vi "GetRectangles.vi"(0 "reference in":refnum<class "Pgui_Obj.lvclass">, 5 "error in (no error)":errorcluster) -> (14 "reference out":refnum<class "Pgui_Obj.lvclass">, 15 "Rectangles":string, 19 "error out":errorcluster)   [LabVIEW 2019, in "Pgui_Obj.lvclass"]
uses:
  Pgui_Obj.lvclass
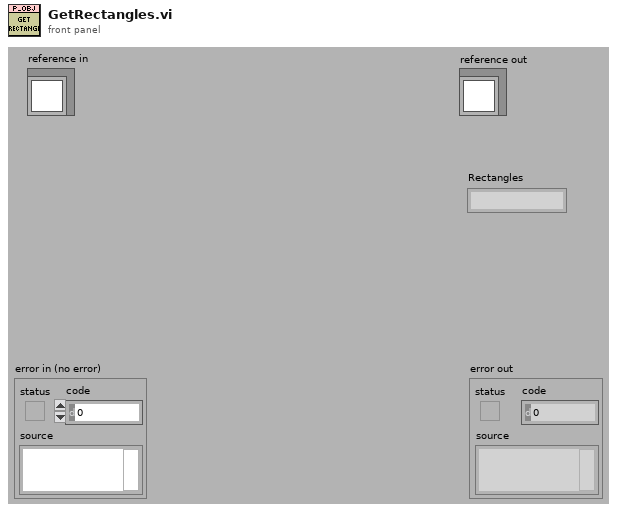
[diagram p1: front panel]
types:
  T1 = typedef "Pgui_Obj.lvclass/ObjectAttributes.ctl" = cluster{"Children":refnum<class "Pgui_Obj.lvclass">[], "Draw Instr":picture, "Params":cluster{"left":i16, "top":i16, "right":i16, "bottom":i16}, "Parent_Pgui_Obj":refnum<class "Pgui_Obj.lvclass">, "MouseOver":bool}
  T2 = cluster{"left":i16, "top":i16, "right":i16, "bottom":i16}
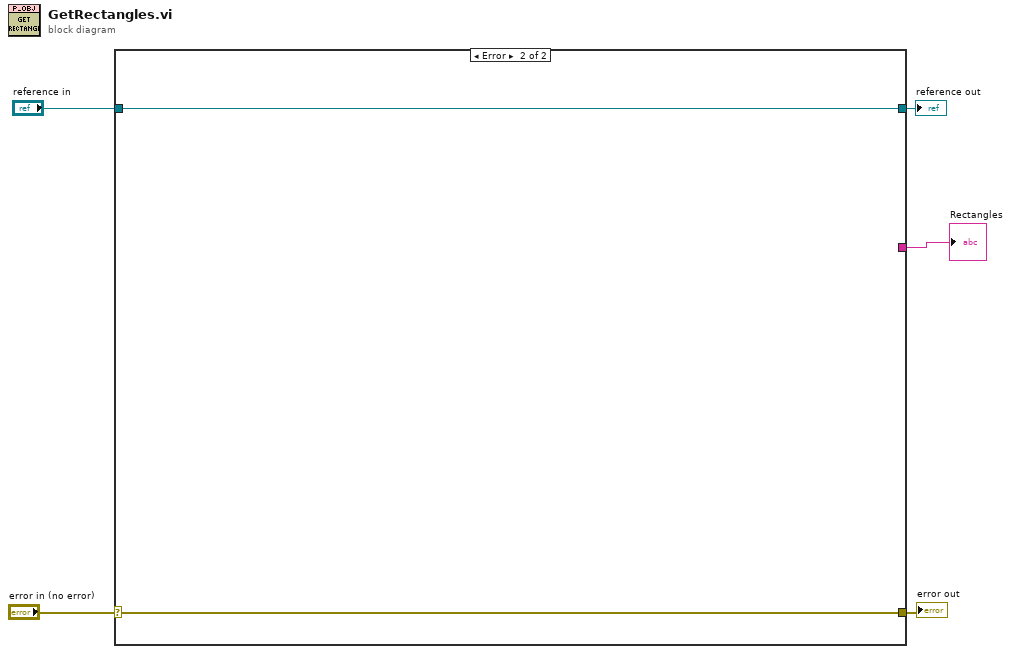
[diagram p0: block diagram]
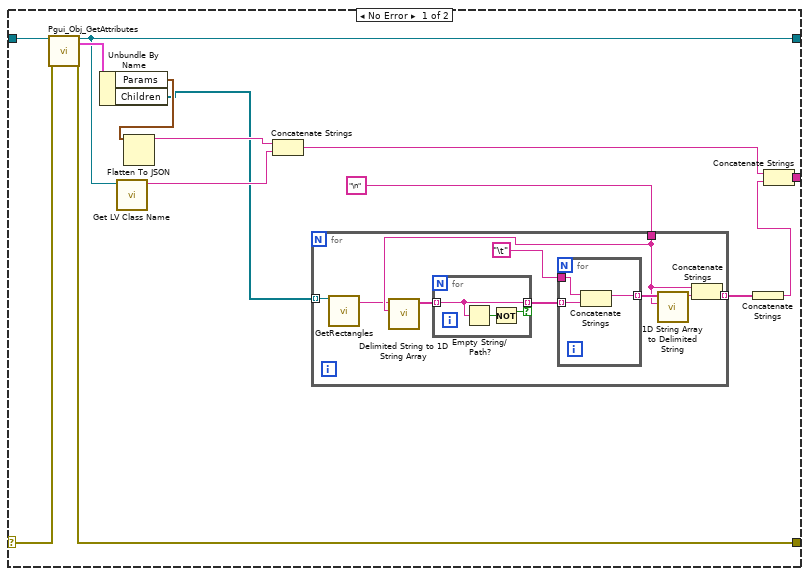
[diagram p2: hidden frame]
diagram:
  n1 = case shown="Error" "error in (no error)" {
    selector: "error in (no error)" -> [w19 w36]
    tunnel: [w17 w36] -> w4
    tunnel: [w8 w35] -> w2
    tunnel: "reference in" -> [w16 w35]
    tunnel: [w6 _] -> w1
    frame No Error {
      n2 = call "Pgui_Obj_GetAttributes.vi"("reference in"=w16, "error in (no error)"=w19) -> ("reference out"=w8:refnum<class "Pgui_Obj.lvclass">, "Data"=w18:T1, "error out"=w17:errorcluster)  [unwired: 14 in, 1 out]
      n3 = Unbundle By Name(w18) -> ("Params"=w9:T2, "Children"=w7:refnum<class "Pgui_Obj.lvclass">[])
      n4 = call <vilib>:"Get LV Class Name.vi"("object"=w8) -> ("class name"=w12:string)  [unwired: 9 in, 1 out]
      n5 = Flatten To JSON(anything=w9) -> (JSON string=w11:string)  [unwired: 2 in, 1 out]
      n6 = Concatenate Strings(w11, w12) -> (w13:string)
      n7 = for {
        tunnel: w7 -> [w21] mode=indexing
        tunnel: [w23] -> w10 mode=indexing
        tunnel: "\n" -> [w22]
        n8 = call-dynamic "GetRectangles.vi"("reference in"=w21) -> ("Rectangles"=w20:string)  [unwired: 16 in, 2 out]
        n9 = call <vilib>:"Delimited String to 1D String Array.vi"("delimiter"=w22, "delimited string"=w20) -> ("string array"=w25:string[])  [unwired: 9 in]
        n10 = for {
          tunnel: w25 -> [w31] mode=indexing
          tunnel: [w31] -> w24 mode=indexing if=w29
          n11 = Empty String/Path?(string/path=w31) -> (empty?=w30:bool)
          n12 = Not(x=w30) -> (.not. x?=w29:bool)
        }
        n13 = for {
          tunnel: w24 -> [w34] mode=indexing
          tunnel: "\t" -> [w33]
          tunnel: [w32] -> w27 mode=indexing
          n14 = Concatenate Strings(w33, w34) -> (w32:string)
        }
        n15 = call <vilib>:"1D String Array to Delimited String.vi"("delimiter"=w22, "string array"=w27) -> ("delimited string"=w26:string)  [unwired: 9 in]
        n16 = Concatenate Strings(w22, w26) -> (w23:string)
      }
      n17 = Concatenate Strings(w10) -> (w14:string)
      n18 = Concatenate Strings(w13, w14) -> (w6:string)
    }
    frame Error {
    }
  }
  "error out" <- w4
  "reference out" <- w2
  "Rectangles" <- w1
